vi "公示节点.vi"(0 "b":dbl, 1 "a":dbl) -> ()   [LabVIEW 2017]
panel:
  out "波形图":dbl[][](graph)
  out "y2":dbl
  out "y1":dbl
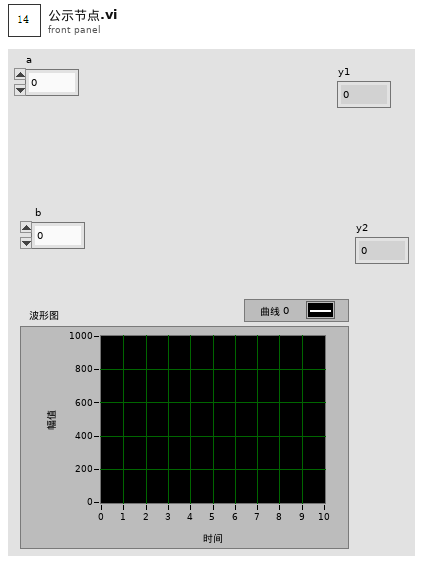
[diagram p1: front panel]
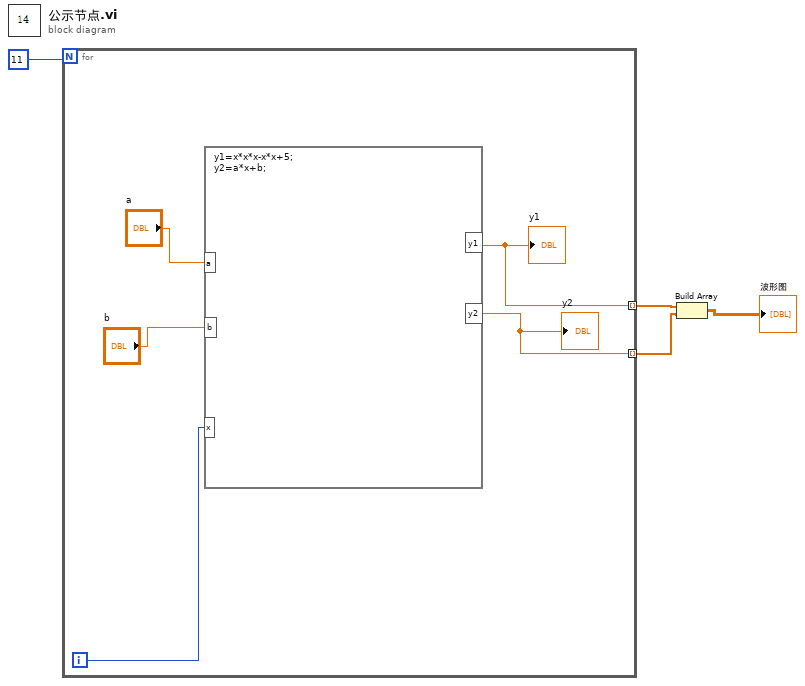
[diagram p0: block diagram]
diagram:
  n1 = for {
    N: 11 -> [_]
    tunnel: [w6] -> w3 mode=indexing
    tunnel: [w5] -> w2 mode=indexing
    i -> [w7]
    n2 = formula code="y1=x*x*x-x*x+5;\ny2=a*x+b;"("a"="a", "b"="b", "x"=w7) -> ("y1"=w6:dbl, "y2"=w5:dbl)
    "y1" <- w6
    "y2" <- w5
  }
  n3 = Build Array(w3, w2) -> (→"波形图":dbl[][])
